vi "Save SV to Library.vi"(8 "Error In":errorcluster, 9 "Shared Variables":refnum<k21>[](array[refnum]), 10 "Library Path":path, 11 "CS++DSCManager in":refnum<class "CS++DSCManager.lvclass">) -> (0 "Error Out":errorcluster, 2 "Complete Path":path, 3 "CS++DSCManager out":refnum<class "CS++DSCManager.lvclass">)   [LabVIEW 2016, in "CS++DSCManager.lvlib" / "CS++DSCManager.lvclass"]
doc: "Saves the deployed configuration of shared variables to one or several LabVIEW project libraries."
uses:
  CS++DSCManager.lvclass
  <vilib>/lvdsc/process/SharedVariablesToLib.vi
  <vilib>/lvdsc/NI_DSC.lvlib
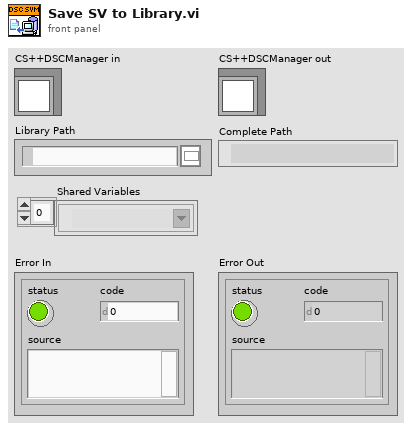
[diagram p1: front panel]
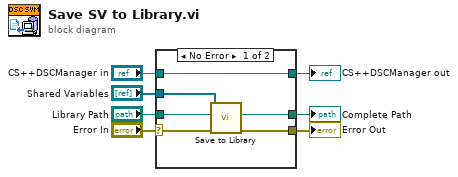
[diagram p0: block diagram]
diagram:
  n1 = case shown="No Error" "Error In" {
    selector: "Error In" -> [w13 w16]
    tunnel: [w10 w16] -> w6
    tunnel: [w11 w15] -> w4
    tunnel: "CS++DSCManager in" -> [w11 w15]
    tunnel: "Library Path" -> [w12 w14]
    tunnel: "Shared Variables" -> [w9 _]
    tunnel: [w8 w14] -> w1
    frame No Error {
      n2 = call-poly <vilib>:"Save to Library.vi"("error in (no error)"=w13, "library path"=w12, "shared variables"=w9) -> ("error out"=w10:errorcluster, "complete path"=w8:path)  [unwired: 7 in]
    }
    frame Error {
    }
  }
  "Error Out" <- w6
  "CS++DSCManager out" <- w4
  "Complete Path" <- w1
